vi "HEWH RLT Compile TCs For Station.vi"(8 "Error In":errorcluster, 9 "Station ID":string="A", 10 "Agilent Cluster Array In":T1[](array[typedef])=[{"Label"="T1-17", "Agilent Channel"="109", "Panel ID"="", "Source"="", "Temperature"=20.0}, {"Label"="T1-18", "Agilent Channel"="110", "Panel ID"="", "Source"="", "Temperature"=21.0}], 11 "RLT Station Channels In":T2={"MW100"={"Station A Channels, MW100"=[], "Station B Channels, MW100"=[], "Station C Channels, MW100"=[], "Station D Channels, MW100"=[]}, "Agilent"={"Station A Channels, Agilent"=[["T1-17", "109"], ["T1-18", "110"]], "Station B Channels, Agilent"=[], "Station C Channels, Agilent"=[], "Station D Channels, Agilent"=[]}}) -> (0 "Error Out":errorcluster, 2 "Agilent Cluster Array Out":T1[](array[typedef])=[{"Label"="T1-17", "Agilent Channel"="109", "Panel ID"="", "Source"="", "Temperature"=20.0}, {"Label"="T1-18", "Agilent Channel"="110", "Panel ID"="", "Source"="", "Temperature"=21.0}], 3 "RLT Station Channels Out":T2={"MW100"={"Station A Channels, MW100"=[], "Station B Channels, MW100"=[], "Station C Channels, MW100"=[], "Station D Channels, MW100"=[]}, "Agilent"={"Station A Channels, Agilent"=[["T1-17", "109"], ["T1-18", "110"]], "Station B Channels, Agilent"=[], "Station C Channels, Agilent"=[], "Station D Channels, Agilent"=[]}}, 5 "Data (Label,Data)":string[][](array[string])=[["T1-17", "20.000000"], ["T1-18", "21.000000"]])   [LabVIEW 2016]
uses:
  Type Definitions/HEWH Agilent Cluster.ctl
  Type Definitions/HEWH RLT MW100 Station Channels.ctl
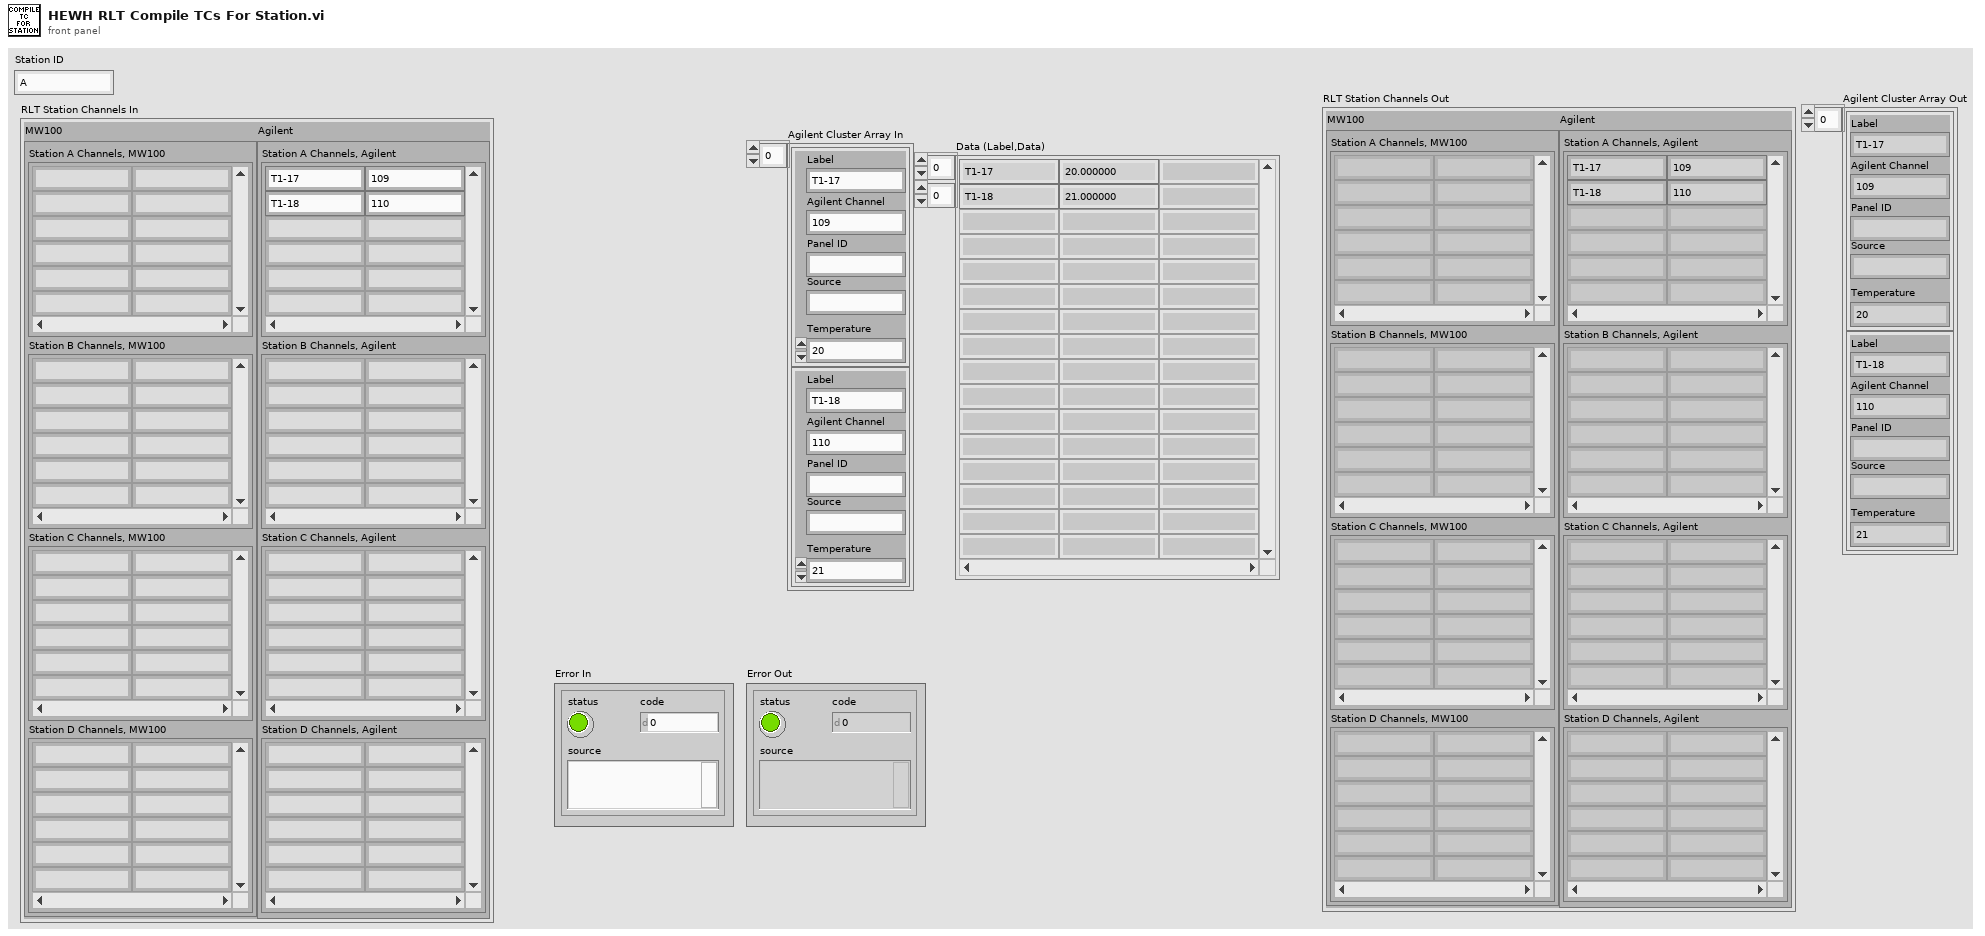
[diagram p1: front panel]
types:
  T1 = typedef "HEWH Agilent Cluster.ctl" = cluster{"Label":string, "Agilent Channel":string, "Panel ID":string, "Source":string, "Temperature":dbl}
  T2 = typedef "HEWH RLT MW100 Station Channels.ctl" = cluster{"MW100":cluster{"Station A Channels, MW100":string[][], "Station B Channels, MW100":string[][], "Station C Channels, MW100":string[][], "Station D Channels, MW100":string[][]}, "Agilent":cluster{"Station A Channels, Agilent":string[][], "Station B Channels, Agilent":string[][], "Station C Channels, Agilent":string[][], "Station D Channels, Agilent":string[][]}}
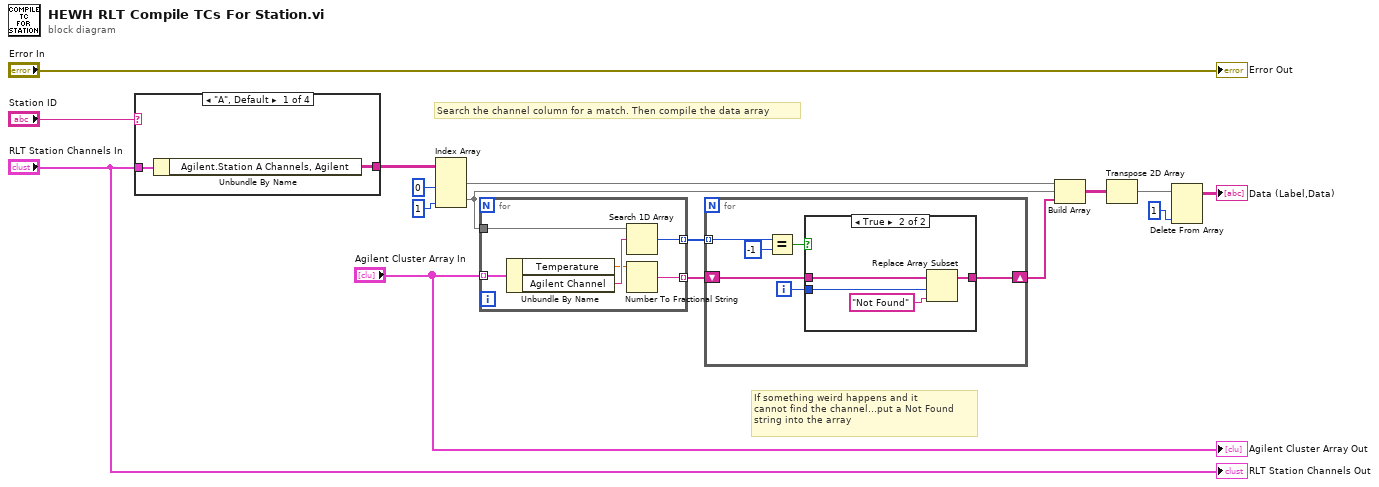
[diagram p0: block diagram]
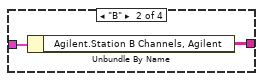
[diagram p2: hidden frame]
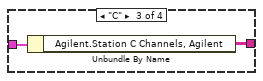
[diagram p3: hidden frame]
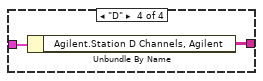
[diagram p4: hidden frame]
diagram:
  # "If something weird happens and it \ncannot find the channel...put a Not Found\nstring into the array"
  # "Search the channel column for a match. Then compile the data array"
  n1 = case shown="\"A\", Default" "Station ID" {
    tunnel: "RLT Station Channels In" -> [w18 w20 w22 w24]
    tunnel: [w17 w19 w21 w23] -> w4
    frame "A", Default {
      n2 = Unbundle By Name(w18) -> ("Agilent.Station A Channels, Agilent"=w17:string[][])
    }
    frame "B" {
      n3 = Unbundle By Name(w20) -> ("Agilent.Station B Channels, Agilent"=w19:string[][])
    }
    frame "C" {
      n4 = Unbundle By Name(w22) -> ("Agilent.Station C Channels, Agilent"=w21:string[][])
    }
    frame "D" {
      n5 = Unbundle By Name(w24) -> ("Agilent.Station D Channels, Agilent"=w23:string[][])
    }
  }
  n6 = Index Array(array=w4, index (col) #1=0 ("disabled index (col)"), index (col) #2=1 ("disabled index (col)")) -> (element #1=w8:string[], element #2=w7:string[])  [unwired: 2 in]
  n7 = for {
    tunnel: "Agilent Cluster Array In" -> [w30] mode=indexing
    tunnel: w7 -> [w29]
    tunnel: [w27] -> w13 mode=indexing
    tunnel: [w26] -> w12 mode=indexing
    n8 = Unbundle By Name(w30) -> ("Temperature"=w25:dbl, "Agilent Channel"=w28:string)
    n9 = Search 1D Array(1D array=w29, element=w28) -> (index of element=w27:i32)  [unwired: 1 in]
    n10 = Number To Fractional String(number=w25) -> (F-format string=w26:string)  [unwired: 3 in]
  }
  n11 = for {
    tunnel: w13 -> [w36] mode=indexing
    shift-right: [w31] -> w11
    shift-left: w12 -> [w33]
    i -> [w32]
    n12 = Equal?(x=w36, y=-1) -> (x = y?=w34:bool)
    n13 = case shown="True" w34 {
      tunnel: w33 -> [w37 w41]
      tunnel: w32 -> [_ w39]
      tunnel: [w37 w38] -> w31
      frame False {
      }
      frame True {
        n14 = Replace Array Subset(array=w41, new element="Not Found", index=w39) -> (w38:string[])
      }
    }
  }
  n15 = Build Array(w8, w7, w11) -> (w14:string[][])
  n16 = Transpose 2D Array(2D array=w14) -> (transposed array=w3:string[][])
  n17 = Delete From Array(array=w3, index (col)=1 ("index (row)")) -> (array with subset deleted=→"Data (Label,Data)":string[][])  [unwired: 2 in, 1 out]
  "Error Out" <- "Error In"
  "RLT Station Channels Out" <- "RLT Station Channels In"
  "Agilent Cluster Array Out" <- "Agilent Cluster Array In"
